vi "cal_end_time.vi"(9 "恒温时间":i32, 10 "分钟":i32, 11 "小时":i32) -> (2 "结束分钟":i32, 3 "结束小时":i32)   [LabVIEW 2017]
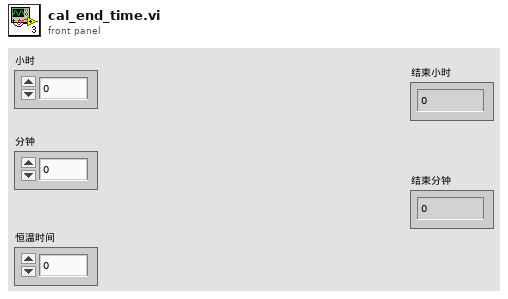
[diagram p1: front panel]
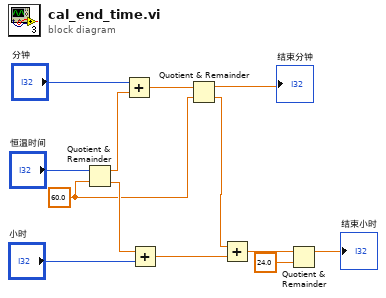
[diagram p0: block diagram]
diagram:
  w7 = 60.0 ("y")
  n1 = Quotient & Remainder(x="恒温时间", y=w7) -> (x-y*floor(x/y)=w10:dbl, floor(x/y)=w12:dbl)
  n2 = Add(x="分钟", y=w10) -> (x+y=w8:dbl)
  n3 = Add(x=w12, y="小时") -> (x+y=w6:dbl)
  n4 = Quotient & Remainder(x=w8, y=w7) -> (x-y*floor(x/y)=→"结束分钟":dbl, floor(x/y)=w5:dbl)
  n5 = Add(x=w5, y=w6) -> (x+y=w4:dbl)
  n6 = Quotient & Remainder(x=w4, y=24.0) -> (x-y*floor(x/y)=→"结束小时":dbl)  [unwired: 1 out]
